vi "ACT_Loop.vi"() -> ()   [LabVIEW 2020, in "Cone_Stabber_ACT.lvlib"]
uses:
  ConeStabber/Cone_Stabber_ACT.lvlib
  Cluster_CMD_ACT_Data.ctl
  ConeStabber/ENUM_CMD_Cone_Stabber_Mode select.ctl
  ENUM_ACT_State.ctl
  <vilib>/Rock Robotics/WPI/MotorControl/WPI_MotorControlDeviceRef.ctl
  <vilib>/Rock Robotics/WPI/MotorControl/WPI_MotorControlType.ctl
  <vilib>/Rock Robotics/SystemInterfaces/DIO/FPGA_DIOPWMChannel.ctl
  <vilib>/Rock Robotics/WPI/PWM/WPI_PWMDeadband.ctl
  <vilib>/Rock Robotics/SystemInterfaces/DIO/FPGA_DIOChannel.ctl
  <vilib>/Rock Robotics/WPI/ThirdParty/Phoenix-LabVIEW/Motor Controller/Controls/CTRE_Phoenix_MotorControl_ControlMode.ctl
  ENUM_ACT_Action.ctl
  Utility/Global_STOP.vi
  Global_CMD_ACT_Data In.vi
  Global_ACT_Data Out.vi
panel:
  out "Input DBL Data":T1
  out "Motor Value":dbl
  out "Cycle Time (S)":dbl format="%.3g"
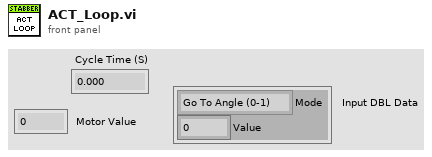
[diagram p1: front panel]
types:
  T1 = typedef "Cone_Stabber_ACT.lvlib/Cluster_CMD_ACT_Data.ctl" = cluster{"Mode":T2, "Value":dbl}
  T2 = typedef "Cone_Stabber_ACT.lvlib/ENUM_CMD_Cone_Stabber_Mode select.ctl" = enum16{"Go To Angle (0-1)", "Stop"}
  T3 = typedef "CTRE_Phoenix_MotorControl_ControlMode.ctl" = u16
  T4 = typedef "WPI_MotorControlDeviceRef.ctl" = cluster{"DeviceStatus":errorcluster, "Type":T5, "PWM":cluster{"PWM Channel":T6, "DeadBand":T7}, "CAN":cluster{"Device Number":u8, "SetOutput VI Ref":variant, "GetOutput VI Ref":variant, "Enable VI Ref":variant, "Disable VI Ref":variant, "Data":variant}, "Invert":bool, "DIO PWM":cluster{"PWM \"Enable\" Channel":T6, "DIOChannel":T8, "PWM Rate":dbl}}
  T5 = typedef "WPI_MotorControlType.ctl" = enum16{"PWM", "CAN", "DIO PWM"}
  T6 = typedef "FPGA_DIOPWMChannel.ctl" = enum8{"PWM 0", "PWM 1", "PWM 2", "PWM 3", "PWM 4", "PWM 5", "PWM 6", "PWM 7", "PWM 8", "PWM 9", "PWM MXP 0", "PWM MXP 1", "PWM MXP 2", "PWM MXP 3", "PWM MXP 4", "PWM MXP 5", "PWM MXP 6", "PWM MXP 7", "PWM MXP 8", "PWM MXP 9", "Invalid"}
  T7 = typedef "WPI_PWMDeadband.ctl" = cluster{"Name":string, "maxPositivePwm":i32, "minPositivePwm":i32, "centerPwm":i32, "maxNegativePwm":i32, "minNegativePwm":i32, "angularRange":u16}
  T8 = typedef "FPGA_DIOChannel.ctl" = enum8{"DIO 0", "DIO 1", "DIO 2", "DIO 3", "DIO 4", "DIO 5", "DIO 6", "DIO 7", "DIO 8", "DIO 9", "DIO MXP 0", "DIO MXP 1", "DIO MXP 2", "DIO MXP 3", "DIO MXP 4", "DIO MXP 5", "DIO MXP 6", "DIO MXP 7", "DIO MXP 8", "DIO MXP 9", "DIO MXP 10", "DIO MXP 11", "DIO MXP 12", "DIO MXP 13", "DIO MXP 14", "DIO MXP 15", "SPI Port CS1", "SPI Port CS2", "SPI Port CS3", "SPI Port MISO", "SPI Port MOSI", "Invalid"}
  T9 = typedef "Cone_Stabber_ACT.lvlib/ENUM_ACT_State.ctl" = enum16{"Startup", "Going to Angle", "Shutdown"}
  T10 = typedef "Cone_Stabber_ACT.lvlib/ENUM_ACT_Action.ctl" = enum16{"Config Motor", "No Action", "Reset Time", "Reset All", "Set Angle", "Stop"}
  T11 = cluster{"ConeStabberMotor":T4, "State":T9, "Previous State":T9, "Current Time":timestamp, "Previous Time":timestamp, "Start Time":timestamp, "Target Time (ms)":u32, "Cycle Time(S)":dbl, "ACT Input":T1, "Motor Value":dbl, "Control Mode":T3}
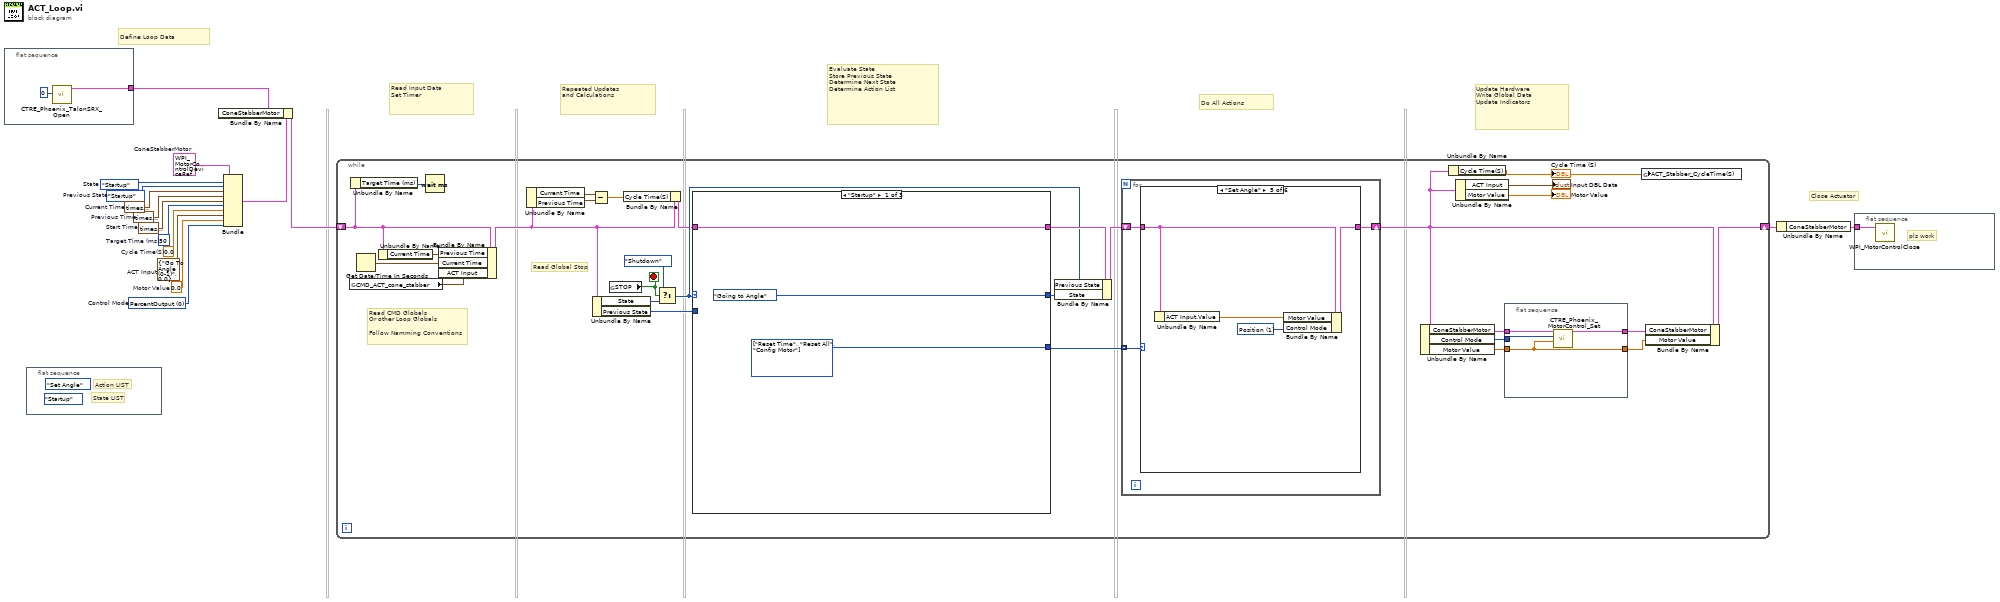
[diagram p0: block diagram]
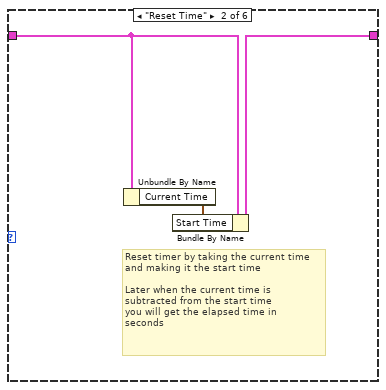
[diagram p3: hidden frame]
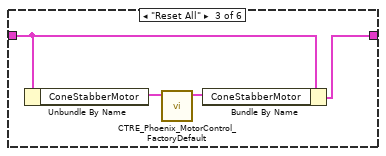
[diagram p4: hidden frame]
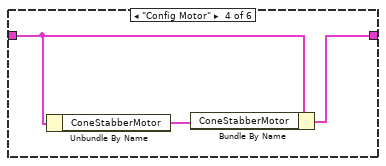
[diagram p5: hidden frame]
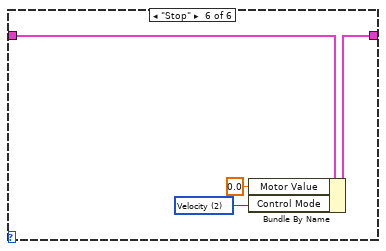
[diagram p6: hidden frame]
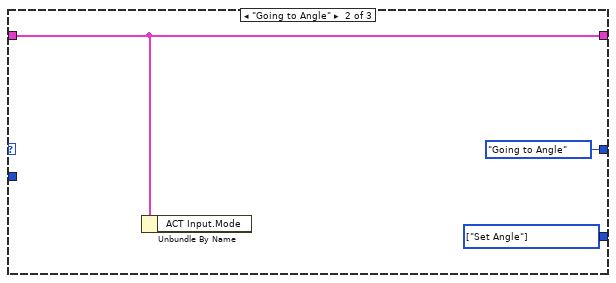
[diagram p7: hidden frame]
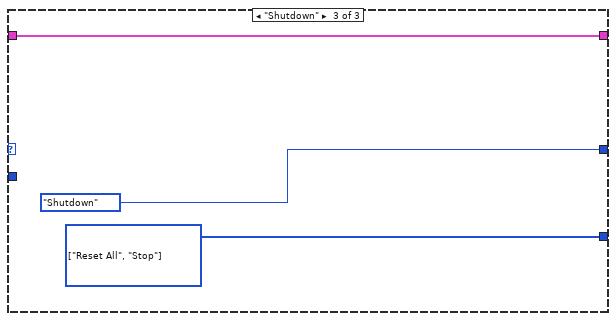
[diagram p8: hidden frame]
diagram:
  w1 = T3 0 items=["PercentOutput"=0, "Position"=1, "Velocity"=2, "Current"=3, "Follower"=5, "MotionProfile"=6, "MotionMagic"=7, "MotionProfileArc"=10, "Disabled"=15]  # Control Mode
  w3 = T4 {"DeviceStatus"={"status"=FALSE, "code"=0, "source"=""}, "Type"=enum."PWM", "PWM"={"PWM Channel"=enum."PWM 1", "DeadBand"={"Name"="", "maxPositivePwm"=0, "minPositivePwm"=0, "centerPwm"=0, "maxNegativePwm"=0, "minNegativePwm"=0, "angularRange"=0}}, "CAN"={"Device Number"=0, "SetOutput VI Ref"=variant(enum8{"Percent VBus", "Current", "Speed", "Position", "Voltage"} enum."Percent VBus"), "GetOutput VI Ref"=variant(refnum<k1> refnum), "Enable VI Ref"=variant(dbl 12.0), "Disable VI Ref"=variant(enum8{"Percent VBus", "Speed", "Position", "Slave", "Unchanged / Invalid", "Voltage Compensation", "Current", "Motion Profile"} enum."Percent VBus"), "Data"=variant}, "Invert"=FALSE, "DIO PWM"={"PWM \"Enable\" Channel"=enum."Invalid", "DIOChannel"=enum."Invalid", "PWM Rate"=0.0}}  # ConeStabberMotor
  w8 = 0.0  # Cycle Time(S)
  w9 = ENUM_ACT_State."Startup"  # Previous State
  w10 = timestamp(0 s since 1904-01-01)  # Previous Time
  w11 = u32 50  # Target Time (ms)
  w12 = 0.0  # Motor Value
  w13 = T1 {"Mode"=enum."Go To Angle (0-1)", "Value"=0.0}  # ACT Input
  w14 = timestamp(0 s since 1904-01-01)  # Start Time
  w15 = timestamp(0 s since 1904-01-01)  # Current Time
  w16 = ENUM_ACT_State."Startup"  # State
  # "Close Actuator"
  # "Define Loop Data"
  # "Repeated Updates\nand Calculations"
  # "Read Input Data\nSet Timer"
  # "Evaluate State\nStore Previous State\nDetermine Next State\nDetermine Action List"
  # "Do All Actions"
  # "Update Hardware\nWrite Global Data\nUpdate Indicators"
  n1 = flat-sequence {
    tunnel: [w17] -> w2
    frame #0 {
      n2 = call <vilib>:"CTRE_Phoenix_TalonSRX_Open.vi"("Device Number"=u8 0) -> ("PhoenixMotorControlDevRef"=w17:T4)  [unwired: 9 in, 1 out]
    }
  }
  n3 = flat-sequence {
    frame #0 {
      (unwired) ENUM_ACT_State."Startup" ("State")
      (unwired) ENUM_ACT_Action."Set Angle" ("Action")
      # "State LIST"
      # "Action LIST"
    }
  }
  n4 = Bundle("ConeStabberMotor"=w3, "State"=w16, "Previous State"=w9, "Current Time"=w15, "Previous Time"=w10, "Start Time"=w14, "Target Time (ms)"=w11, "Cycle Time(S)"=w8, "ACT Input"=w13, "Motor Value"=w12, "Control Mode"=w1) -> (w5:T11)  [unwired: 1 in]
  n5 = Bundle By Name(cluster=w5, "ConeStabberMotor"=w2) -> (w4:T11)
  n6 = while {
    shift-right: [w23] -> w6
    shift-left: w4 -> [w38]
    stop <- w43 stop-if-true
    # "Read CMD Globals\nOr other Loop Globals\n\nFollow Namming Conventions"
    # "Read Global Stop"
    n7 = global read "Global_CMD_ACT_Data In.vi" "CMD_ACT_cone_stabber"() -> (w27:T1)
    n8 = Unbundle By Name(w38) -> ("Target Time (ms)"=w40:u32)
    n9 = Get Date/Time In Seconds() -> (seconds since 1Jan1904=w47:timestamp)
    n10 = Unbundle By Name(w38) -> ("Current Time"=w39:timestamp)
    n11 = Wait (ms)(milliseconds to wait=w40) -> ()  [unwired: 1 out]
    n12 = Bundle By Name(cluster=w38, "Previous Time"=w39, "Current Time"=w47, "ACT Input"=w27) -> (w32:T11)
    n13 = Unbundle By Name(w32) -> ("Current Time"=w33:timestamp, "Previous Time"=w34:timestamp)
    n14 = Subtract(x=w33, y=w34) -> (x-y=w30:dbl)
    n15 = Unbundle By Name(w32) -> ("State"=w41:T9, "Previous State"=w37:T9)
    n16 = global read "Global_STOP.vi" "STOP"() -> (w43:bool)
    n17 = Bundle By Name(cluster=w32, "Cycle Time(S)"=w30) -> (w31:T11)
    n18 = Select(t=ENUM_ACT_State."Shutdown" ("State"), s=w43, f=w41) -> (s? t:f=w35:T9)
    n19 = case shown="\"Startup\"" w35 {
      tunnel: w31 -> [w76 w79 w82]
      tunnel: [w76 w79 w82] -> w45
      tunnel: [ENUM_ACT_State."Going to Angle" ("State") ENUM_ACT_State."Going to Angle" ("State") ENUM_ACT_State."Shutdown" ("State")] -> w44
      tunnel: [w75 w77 w80] -> w29
      tunnel: w37 -> [_ _ _]
      frame "Startup" {
        w75 = T10[] [enum."Reset Time", enum."Reset All", enum."Config Motor"] items=["Config Motor", "No Action", "Reset Time", "Reset All", "Set Angle", "Stop"] ("Actions")
      }
      frame "Going to Angle" {
        w77 = T10[] [enum."Set Angle"] items=["Config Motor", "No Action", "Reset Time", "Reset All", "Set Angle", "Stop"] ("Actions")
        n20 = Unbundle By Name(w79) -> ()  [unwired: 1 out]
      }
      frame "Shutdown" {
        w80 = T10[] [enum."Reset All", enum."Stop"] items=["Config Motor", "No Action", "Reset Time", "Reset All", "Set Angle", "Stop"] ("Actions")
      }
    }
    n21 = Bundle By Name(cluster=w45, "Previous State"=w35, "State"=w44) -> (w46:T11)
    n22 = for {
      tunnel: w29 -> [w54] mode=indexing
      shift-right: [w53] -> w24
      shift-left: w46 -> [w52]
      n23 = case shown="\"Set Angle\"" w54 {
        tunnel: w52 -> [w55 w58 w60 w64 w69 w73]
        tunnel: [w55 w57 w59 w63 w68 w72] -> w53
        frame "No Action" {
        }
        frame "Reset Time" {
          # "Reset timer by taking the current time\nand making it the start time\n\nLater when the current time is \nsubtracted from the start time\nyou will get the elapsed time in \nseconds"
          n24 = Unbundle By Name(w58) -> ("Current Time"=w56:timestamp)
          n25 = Bundle By Name(cluster=w58, "Start Time"=w56) -> (w57:T11)
        }
        frame "Reset All" {
          n26 = Unbundle By Name(w60) -> ("ConeStabberMotor"=w62:T4)
          n27 = call <vilib>:"CTRE_Phoenix_MotorControl_FactoryDefault.vi"("PhoenixMotorControlDevRef"=w62) -> ("PhoenixMotorControlDevRef"=w61:T4)  [unwired: 9 in, 1 out]
          n28 = Bundle By Name(cluster=w60, "ConeStabberMotor"=w61) -> (w59:T11)
        }
        frame "Config Motor" {
          n29 = Unbundle By Name(w64) -> ("ConeStabberMotor"=w65:T4)
          n30 = Bundle By Name(cluster=w64, "ConeStabberMotor"=w65) -> (w63:T11)
        }
        frame "Set Angle" {
          w67 = T3 1 items=["PercentOutput"=0, "Position"=1, "Velocity"=2, "Current"=3, "Follower"=5, "MotionProfile"=6, "MotionMagic"=7, "MotionProfileArc"=10, "Disabled"=15] ("Control Mode")
          n31 = Unbundle By Name(w69) -> ("ACT Input.Value"=w66:dbl)
          n32 = Bundle By Name(cluster=w69, "Motor Value"=w66, "Control Mode"=w67) -> (w68:T11)
        }
        frame "Stop" {
          w70 = T3 2 items=["PercentOutput"=0, "Position"=1, "Velocity"=2, "Current"=3, "Follower"=5, "MotionProfile"=6, "MotionMagic"=7, "MotionProfileArc"=10, "Disabled"=15] ("Control Mode")
          n33 = Bundle By Name(cluster=w73, "Motor Value"=0.0, "Control Mode"=w70) -> (w72:T11)
        }
      }
    }
    n34 = Unbundle By Name(w24) -> ("ConeStabberMotor"=w26:T4, "Control Mode"=w21:T3, "Motor Value"=w20:dbl)
    n35 = Unbundle By Name(w24) -> ("Cycle Time(S)"=w22:dbl)
    "Cycle Time (S)" <- w22
    n36 = Unbundle By Name(w24) -> ("ACT Input"=→"Input DBL Data":T1, "Motor Value"=→"Motor Value":dbl)
    n37 = flat-sequence {
      tunnel: w26 -> [w51]
      tunnel: [w50] -> w25
      tunnel: w21 -> [w49]
      tunnel: w20 -> [w48]
      tunnel: [w48] -> w19
      frame #0 {
        n38 = call <vilib>:"CTRE_Phoenix_MotorControl_Set.vi"("Output"=w48, "Control Mode"=w49, "PhoenixMotorControlDevRef"=w51) -> ("PhoenixMotorControlDevRef"=w50:T4)  [unwired: 7 in, 1 out]
      }
    }
    n39 = global write "Global_ACT_Data Out.vi" "ACT_Stabber_CycleTime(S)"(w22) -> ()
    n40 = Bundle By Name(cluster=w24, "ConeStabberMotor"=w25, "Motor Value"=w19) -> (w23:T11)
  }
  n41 = Unbundle By Name(w6) -> ("ConeStabberMotor"=w7:T4)
  n42 = flat-sequence {
    tunnel: w7 -> [w83]
    frame #0 {
      # "pls work"
      n43 = call <vilib>:"WPI_MotorControlClose.vi"("MotorControlDevRef"=w83) -> ()  [unwired: 10 in, 1 out]
    }
  }
